vi "Create Property List.vi"(11 "Channels (1-64)":u16) -> (3 "Property List":string[](array[string]))   [LabVIEW 2020, in "slsc-switch-benchmarks.lvlib"]
uses:
  slsc-switch-benchmarks.lvlib
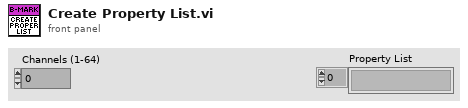
[diagram p1: front panel]
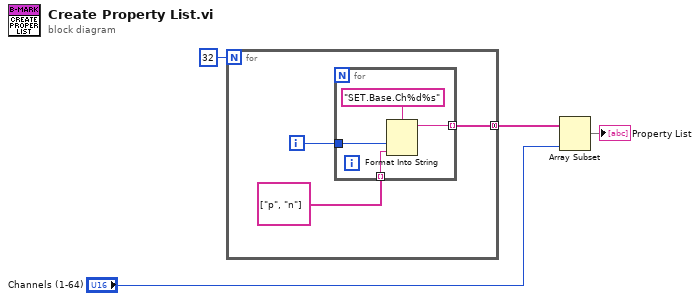
[diagram p0: block diagram]
diagram:
  n1 = for {
    N: 32 -> [_]
    tunnel: [w5] -> w3 mode=concatenating
    i -> [w7]
    n2 = for {
      tunnel: w7 -> [w10]
      tunnel: string[] ["p", "n"] -> [w9] mode=indexing
      tunnel: [w8] -> w5 mode=indexing
      n3 = Format Into String(format string="SET.Base.Ch%d%s", w10, w9) -> (resulting string=w8:string)  [unwired: 2 in, 1 out]
    }
  }
  n4 = Array Subset(array=w3, length="Channels (1-64)") -> (→"Property List":string[])  [unwired: 1 in]
